vi "readBaseHPSettings.vi"(8 "error in (no error)":errorcluster, 11 "Boot in":refnum<class "Boot.lvclass">) -> (0 "error out":errorcluster, 2 "BaseHardpointSettings":T1, 3 "Boot out":refnum<class "Boot.lvclass">)   [LabVIEW 2016, in "Boot.lvclass"]
uses:
  Boot.lvclass
  DataTypes/Settings/Base/BaseHPSettings.ctl
  DataTypes/Settings/Base/Parts/BaseILCIdentitySettings.ctl
  Common_RT_HPILC/DataTypes/HPTimings.ctl
  DataTypes/General/XYZPosition.ctl
  Boot.lvclass/Boot.ctl
  Settings/Settings/Setting.lvclass
  DataTypes/Settings/M1M3SupportSettings.lvlib
  Common_RT_HPILC/RTHPILC.lvlib
  DataTypes/General/M1M3SupportGeneral.lvlib
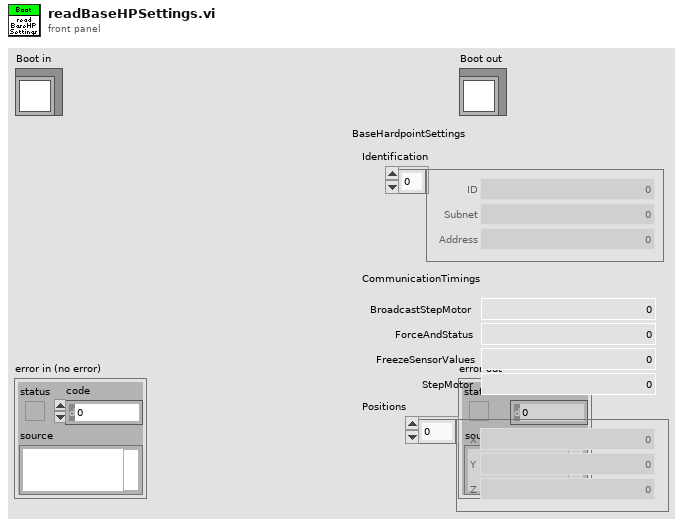
[diagram p1: front panel]
types:
  T1 = typedef "M1M3SupportSettings.lvlib/BaseHPSettings.ctl" = cluster{"Identification":T2[], "CommunicationTimings":T3, "Positions":T4[]}
  T2 = typedef "M1M3SupportSettings.lvlib/BaseILCIdentitySettings.ctl" = cluster{"Subnet":u8, "Address":u8, "ID":i16}
  T3 = typedef "RTHPILC.lvlib/HPTimings.ctl" = cluster{"BroadcastStepMotor":u32, "ForceAndStatus":u32, "FreezeSensorValues":u32, "StepMotor":u32}
  T4 = typedef "M1M3SupportGeneral.lvlib/XYZPosition.ctl" = cluster{"X":sgl, "Y":sgl, "Z":sgl}
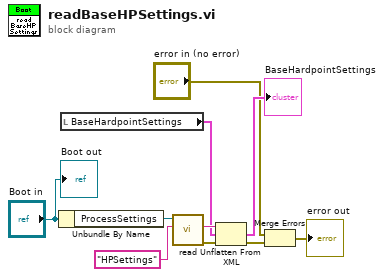
[diagram p0: block diagram]
diagram:
  n1 = Unbundle By Name("Boot in") -> ("ProcessSettings"=w10:refnum<class "Setting.lvclass">)
  n2 = local read "BaseHardpointSettings"() -> (w7:T1)
  n3 = call-dynamic "read.vi"("Name"="HPSettings", "BaseSetting in"=w10) -> ("error out"=w4:errorcluster, "XML"=w8:string)  [unwired: 6 in, 2 out]
  n4 = Unflatten From XML(xml string=w8, type=w7, error in (no error)=w4) -> (value=→"BaseHardpointSettings":T1, error out=w1:errorcluster)
  n5 = Merge Errors("error in (no error)", w1) -> (→"error out":errorcluster)
  "Boot out" <- "Boot in"
